vi "Curtin1_AppendNotes.vi"(11 "Settings":T1={"Name of test"="", "Date"=timestamp(0 s since 1904-01-01), "Location"="", "Template"="", "Soundcard"="", "resolution"=32, "Sampling rate"=48000, "Ch1 Gain "=25.0, "Ch2 Gain"=10.0, "Sample time (s)"=0.3, "Pre-trigger (s)"=0.01, "Hammer Threshold"=10.0, "Positions"=12, "Taps/Position"=5, "Set Names"="", "Freq resolution"=10.0, "Hammer cutoff"=0.0, "Mic cutoff"=0.0, "Double bounce "=0.0, "Hammer Cal"=10.0, "dB Offset"=0.0, "Accel Cal"=10.0, "Vibrometer Cal"=0.0, "Mic Cal"=0.0, "Output"=2, "Voltage Cal"=1.0, "Vibrometer Port"="ASRL27::INSTR", "Range"=4, "High Pass"=2, "Bandwidth"=4, "X Range"=[], "Y Range"=[], "dB Spread"=0.0, "Trigger"=0, "Ch_1"=25, "Ch_2"=25, "flip?"=FALSE, "60Hz"=FALSE, "Time offset"=0.0, "Piezo Cal"=1.0, "Default Notes"=""} {"Ch_2" min=1 step=1; "Ch_1" min=1 max=100 step=1; "Trigger" items=["Hammer (force)", "Self-tap", "Spacebar"]; "Bandwidth" items=["1 kHz"=1, "5 kHz"=5, "10 kHz"=10, "25 kHz"=25, "50 kHz"=50, "100 kHz"=100]; "High Pass" items=["Off", "13 Hz", "104 Hz"]; "Range" items=["10 mm/s"=1, "20 mm/s"=2, "50 mm/s"=5, "100 mm/s"=10, "200 mm/s"=20, "500 mm/s"=50, "1 m/s"=100, "2 m/s"=200]; "Output" items=["Accelerometer", "Speed (from acceleration)", "Microphone", "Vibrometer", "Piezo"]; "Voltage Cal" format="%#_13g"; "Ch2 Gain" format="%#_13g"; "Ch1 Gain" format="%#_13g"; "Double bounce" min=0.0; "Mic cutoff" min=0.0 format="%#_4g"; "Hammer cutoff" min=0.0 format="%#_4g"; "Freq resolution" min=0.0; "Pre-trigger (s)" format="%#_13g"; "Date" format="%<%H:%M\n%d/%m/%y>T"; "resolution" items=["16 bit"=16, "24 bit"=24, "32 bit"=32]; "Sampling rate" items=["22050 samp/s"=22050, "44100 samp/s"=44100, "48000 samp/s"=48000]}) -> (3 "Instrument Notes":string)   [LabVIEW 2022 SP3]
uses:
  PreferencesControl.ctl
  <vilib>/Utility/error.llb/Trim Whitespace One-Sided.vi
panel:
  # "Hz"
  # "dB"
  # "dB"
  # "sec"
  # "sec"
  # "mV/Pa"
  # "mV/m/s2"
  # "mV/mm/s"
  # "V/N"
  # "sec"
  # "sec"
  # "mV/N"
  # "a.u."
  # "a.u."
  # "sec"
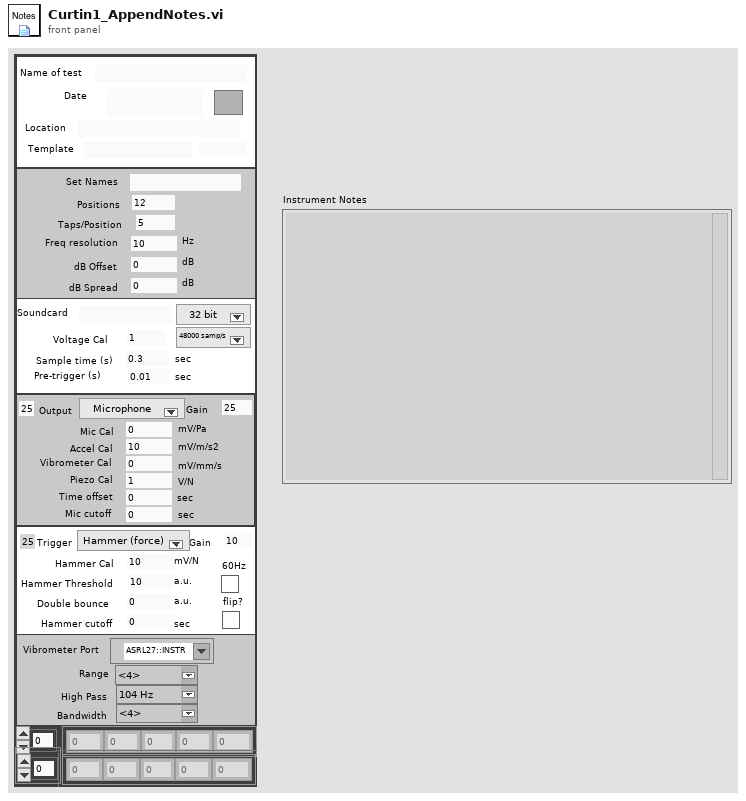
[diagram p1: front panel]
types:
  T1 = typedef "PreferencesControl.ctl" = cluster{"Name of test":string, "Date":timestamp, "Location":string, "Template":string, "Soundcard":string, "resolution":u16, "Sampling rate":u16, "Ch1 Gain ":dbl, "Ch2 Gain":dbl, "Sample time (s)":dbl, "Pre-trigger (s)":dbl, "Hammer Threshold":dbl, "Positions":i16, "Taps/Position":i16, "Set Names":string, "Freq resolution":dbl, "Hammer cutoff":dbl, "Mic cutoff":dbl, "Double bounce ":dbl, "Hammer Cal":dbl, "dB Offset":dbl, "Accel Cal":dbl, "Vibrometer Cal":dbl, "Mic Cal":dbl, "Output":u16, "Voltage Cal":dbl, "Vibrometer Port":refnum<visa-resource-name>, "Range":u16, "High Pass":u16, "Bandwidth":u16, "X Range":cluster{"Minimum":dbl, "Maximum":dbl, "Increment":dbl, "Minor Increment":dbl, "Start":dbl}[], "Y Range":cluster{"Minimum":dbl, "Maximum":dbl, "Increment":dbl, "Minor Increment":dbl, "Start":dbl}[], "dB Spread":dbl, "Trigger":u16, "Ch_1":u8, "Ch_2":u8, "flip?":bool, "60Hz":bool, "Time offset":dbl, "Piezo Cal":dbl, "Default Notes":string}
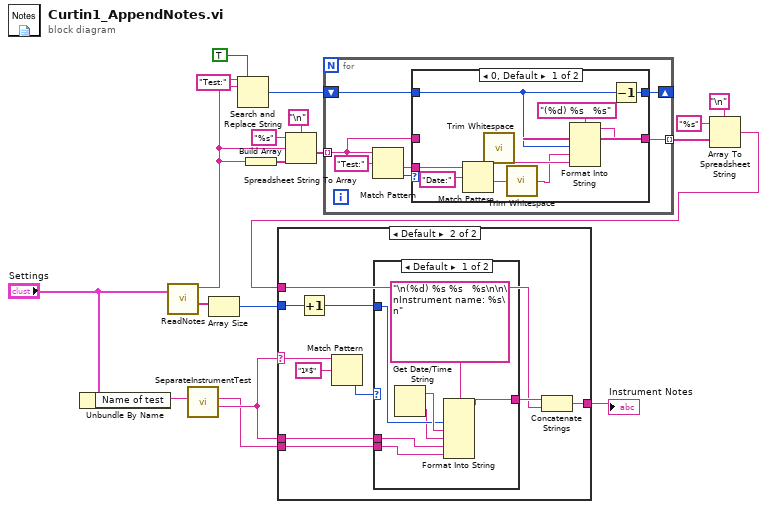
[diagram p0: block diagram]
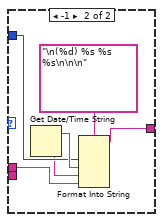
[diagram p4: hidden frame]
diagram:
  n1 = Unbundle By Name("Settings") -> ("Name of test"=w17:string)
  n2 = call "ReadNotes.vi"("Settings"="Settings") -> ("List of Tests"=w14:string[], "Notes"=w2:string)  [unwired: 9 in]
  n3 = call "SeparateInstrumentTest.vi"("Instrument"=w17) -> ("Just test"=w16:string, "Just Instrument"=w15:string)  [unwired: 6 in, 3 out]
  n4 = Array Size(array=w14) -> (size(s)=w13:i32)
  n5 = Search and Replace String(replace all?=TRUE ("replace all? (F)"), input string=w2, search string="Test:" ("regular expression")) -> (number of replacements=w6:i32)  [unwired: 5 in, 3 out]
  n6 = Build Array(w2) -> (w12:string[])
  n7 = Spreadsheet String To Array(delimiter (Tab)="\n", format string="%s", spreadsheet string=w2, array type (2D Dbl)=w12) -> (array=w9:string[])
  n8 = for {
    tunnel: w9 -> [w23] mode=indexing
    tunnel: [w24] -> w5 mode=indexing
    shift-right: [w20] -> _
    shift-left: w6 -> [w21]
    n9 = Match Pattern(string=w23, regular expression="Test:") -> (after substring=w22:string, offset past match=w25:i32)  [unwired: 1 in, 2 out]
    n10 = case shown="0, Default" w25 {
      tunnel: [w27 w38] -> w24
      tunnel: w23 -> [_ w38]
      tunnel: w22 -> [w36 _]
      tunnel: w21 -> [w29 w37]
      tunnel: [w28 w37] -> w20
      frame 0, Default {
        n11 = Match Pattern(string=w36, regular expression="Date:") -> (before substring=w34:string, after substring=w33:string)  [unwired: 1 in, 2 out]
        n12 = call <vilib>:"Trim Whitespace.vi"("string"=w34) -> ("trimmed string"=w31:string)  [unwired: 1 in]
        n13 = call <vilib>:"Trim Whitespace.vi"("string"=w33) -> ("trimmed string"=w30:string)  [unwired: 1 in]
        n14 = Format Into String(format string="(%d) %s   %s", w29, w30, w31) -> (resulting string=w27:string)  [unwired: 2 in, 1 out]
        n15 = Decrement(x=w29) -> (x-1=w28:i32)
      }
      frame -1 {
      }
    }
  }
  n16 = Array To Spreadsheet String(delimiter (Tab)="\n", array=w5, 3:"%s" ("format string")) -> (spreadsheet string=w1:string)
  n17 = case shown="Default" w16 {
    selector: w16 -> [_ w45]
    tunnel: w1 -> [w39 w46]
    tunnel: [w39 w49] -> w19
    tunnel: w16 -> [_ w48]
    tunnel: w15 -> [_ w42]
    tunnel: w13 -> [_ w41]
    frame "" {
    }
    frame Default {
      n18 = Increment(x=w41) -> (x+1=w40:i32)
      n19 = Match Pattern(string=w45, regular expression="1*$") -> (offset past match=w43:i32)  [unwired: 1 in, 3 out]
      n20 = case shown="Default" w43 {
        tunnel: w48 -> [w52 w59]
        tunnel: [w55 w60] -> w47
        tunnel: w42 -> [w51 _]
        tunnel: w40 -> [w53 w58]
        frame Default {
          n21 = Get Date/Time String() -> (date string=w54:string, time string=w50:string)  [unwired: 3 in]
          n22 = Format Into String(format string="\n(%d) %s %s   %s\n\n\nInstrument name: %s\n" ("name or relative path"), w53, w54, w50, w52, w51) -> (resulting string=w55:string)  [unwired: 2 in, 1 out]
        }
        frame -1 {
          n23 = Get Date/Time String() -> (date string=w61:string, time string=w57:string)  [unwired: 3 in]
          n24 = Format Into String(format string="\n(%d) %s %s   %s\n\n\n" ("name or relative path"), w58, w61, w57, w59) -> (resulting string=w60:string)  [unwired: 2 in, 1 out]
        }
      }
      n25 = Concatenate Strings(w47, w46) -> (w49:string)
    }
  }
  "Instrument Notes" <- w19
